vi "AddRows.vi"(6 "GridData":variant, 8 "error in (no error)":errorcluster, 11 "DataGridView in":refnum<class "DataGridView.lvclass">) -> (0 "error out":errorcluster, 3 "DataGridView out":refnum<class "DataGridView.lvclass">)   [LabVIEW 2014, in "DataGridView.lvclass"]
uses:
  DataGridView.lvclass
  DataGridView.lvclass/DataGridView.ctl
  System.Windows.Forms
  GridColumn/GridColumn.lvclass/GridColumn.ctl
  System.Drawing
  GridColumn/Read datatype.vi
  GridColumn/Read Params.vi
  GridColumn/GridColumn.lvclass
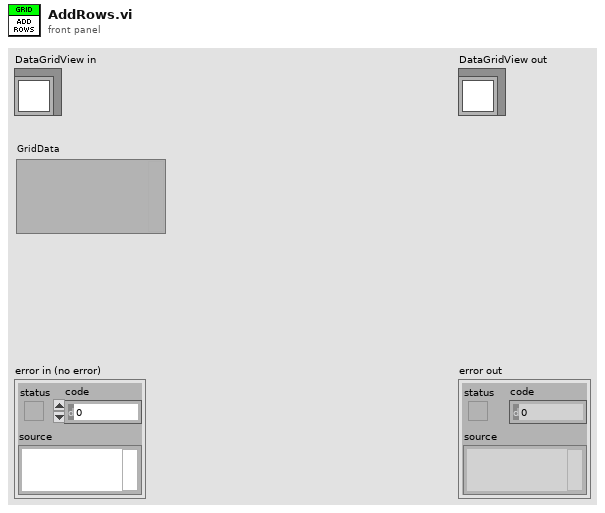
[diagram p1: front panel]
types:
  T1 = enum16{"string", "image", "link", "check", "combo", "button"}
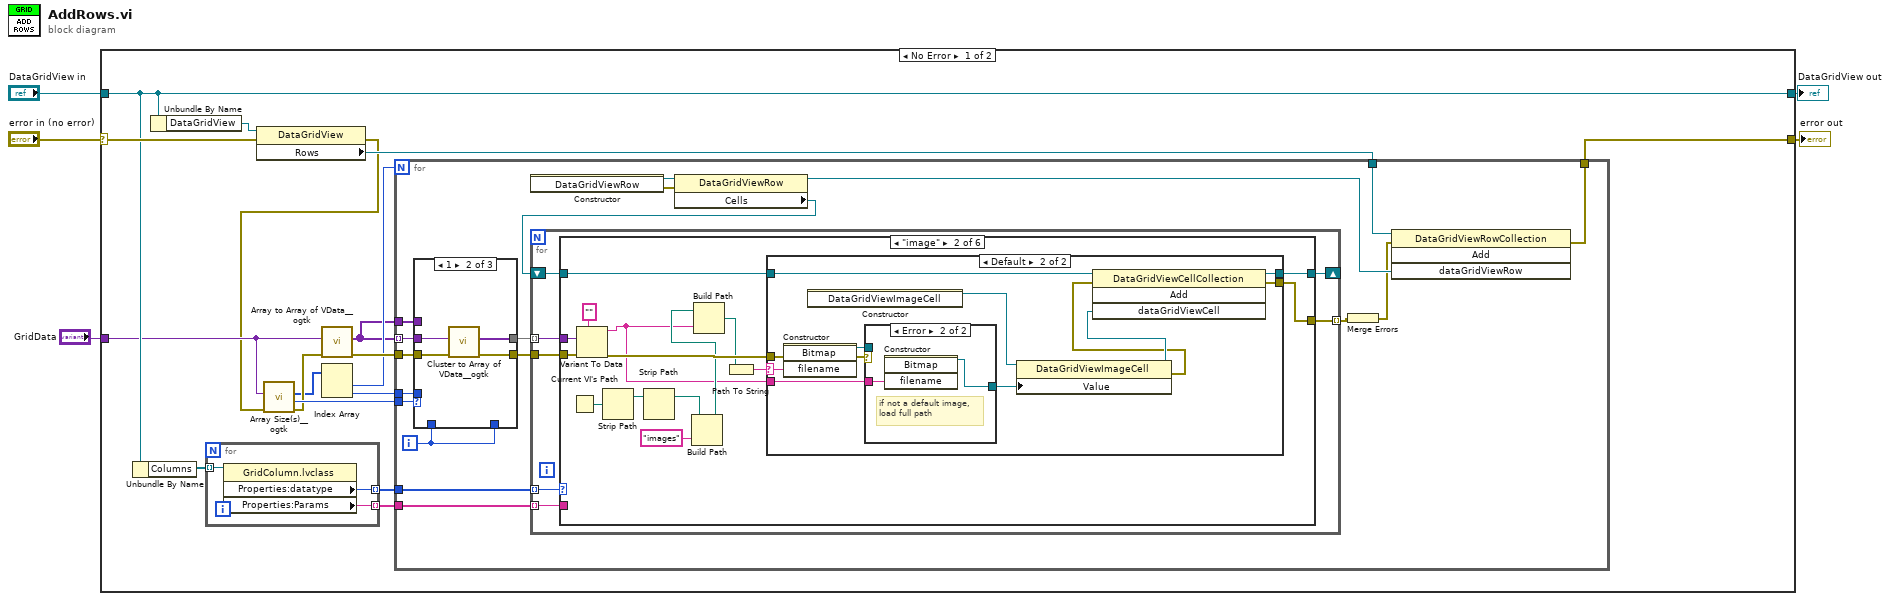
[diagram p0: block diagram]
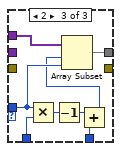
[diagram p3: hidden frame]
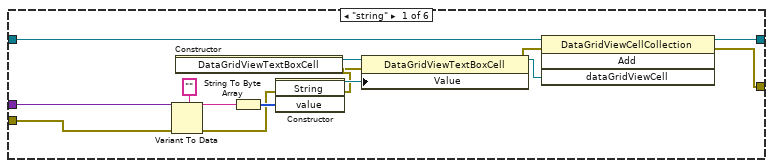
[diagram p4: hidden frame]
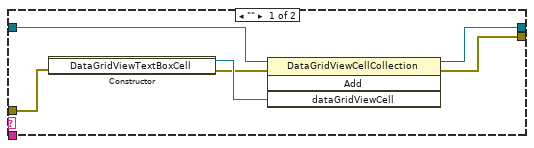
[diagram p5: hidden frame]
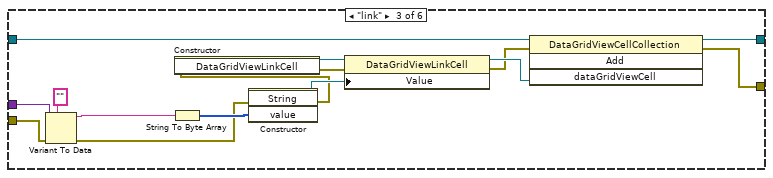
[diagram p7: hidden frame]
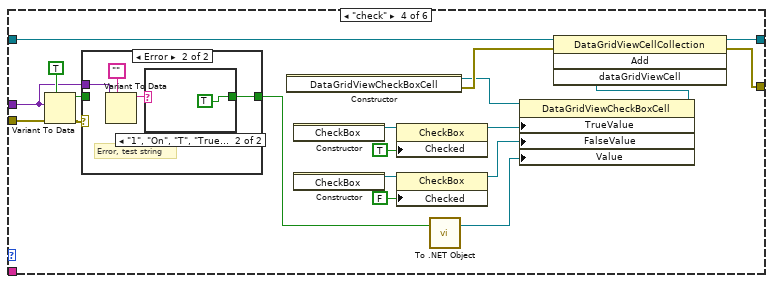
[diagram p8: hidden frame]
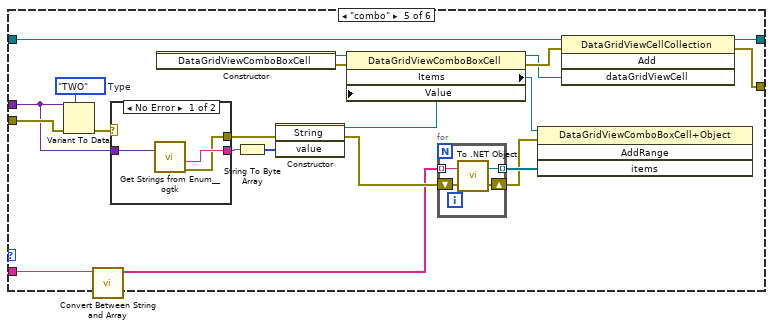
[diagram p11: hidden frame]
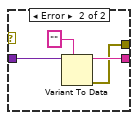
[diagram p12: hidden frame]
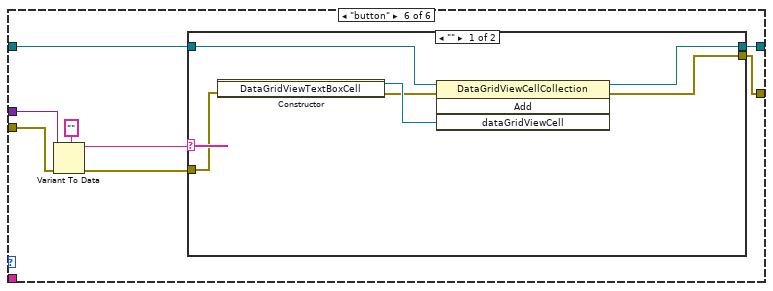
[diagram p13: hidden frame]
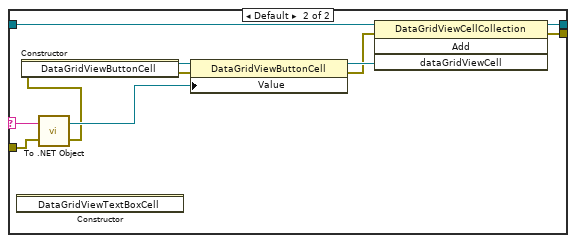
[diagram p14: hidden frame]
diagram:
  n1 = case shown="No Error" "error in (no error)" {
    selector: "error in (no error)" -> [w21 w212]
    tunnel: [w20 w212] -> w4
    tunnel: [w19 w211] -> w2
    tunnel: "DataGridView in" -> [w19 w211]
    tunnel: "GridData" -> [w13 _]
    frame No Error {
      n2 = Unbundle By Name(w19) -> ("Columns"=w18:refnum<class "GridColumn.lvclass">[])
      n3 = Unbundle By Name(w19) -> ("DataGridView"=w22:refnum<k24>)
      n4 = for {
        tunnel: w18 -> [w210] mode=indexing
        tunnel: [w209] -> w17 mode=indexing
        tunnel: [w208] -> w15 mode=indexing
        n5 = property class="GridColumn.lvclass"(reference=w210) -> ("Properties:datatype"=w209:T1, "Properties:Params"=w208:string)  [unwired: 1 in, 2 out]
      }
      n6 = property class="DataGridView"(reference=w22, error in=w21) -> (error out=w10:errorcluster, "Rows"=w16:refnum<k24>)  [unwired: 1 out]
      n7 = call <userlib>:"Array Size(s)__ogtk.vi"("error in (no error)"=w10, "Array"=w13) -> ("error out"=w12:errorcluster, "N dims"=w14:u32, "Size(s)"=w9:u32[])  [unwired: 7 in]
      n8 = call <userlib>:"Array to Array of VData__ogtk.vi"("error in (no error)"=w12, "MultiD Array"=w13) -> ("error out"=w11:errorcluster, "1D Array of Variants"=w6:variant[])  [unwired: 8 in]
      n9 = Index Array(array=w9) -> (element #1=w8:u32, element #2=w7:u32)  [unwired: 2 in]
      n10 = for {
        N: w8 -> [_]
        tunnel: [w40] -> w20
        tunnel: w17 -> [w39]
        tunnel: w16 -> [w33]
        tunnel: w15 -> [w32]
        tunnel: w6 -> [w29] mode=indexing
        tunnel: w14 -> [w28]
        tunnel: w11 -> [w26]
        tunnel: w7 -> [w25]
        tunnel: w6 -> [w23]
        i -> [w24]
        n11 = case shown="1" w28 {
          tunnel: [_ w42 _] -> w30
          tunnel: w29 -> [_ w44 _]
          tunnel: [_ w41 w47] -> w27
          tunnel: w26 -> [_ w43 _]
          tunnel: w25 -> [_ _ w52]
          tunnel: w24 -> [_ _ w51]
          tunnel: w24 -> [_ _ w49]
          tunnel: w23 -> [_ _ w46]
          frame Default {
          }
          frame 1 {
            n12 = call <userlib>:"Cluster to Array of VData__ogtk.vi"("error in (no error)"=w43, "Cluster"=w44) -> ("error out"=w42:errorcluster, "Array of VData"=w41:variant[])  [unwired: 8 in]
          }
          frame 2 {
            n13 = Multiply(x=w52, y=w51) -> (x*y=w50:u32)
            n14 = Decrement(x=w50) -> (x-1=w45:u32)
            n15 = Add(x=w45, y=w49) -> (x+y=w48:u32)
            n16 = Array Subset(array=w46, index=w48, length=w52) -> (w47:variant[])
          }
        }
        n17 = constructor class="DataGridViewRow"() -> (reference out=w37:refnum<k24>, error out=w38:errorcluster)  [unwired: 3 in, 1 out]
        n18 = property class="DataGridViewRow"(reference=w37, error in=w38) -> (reference out=w36:refnum<k24>, "Cells"=w31:refnum<k24>)  [unwired: 1 out]
        n19 = for {
          tunnel: w27 -> [w58] mode=indexing
          tunnel: w39 -> [w59] mode=indexing
          shift-right: [w56] -> _
          shift-left: w31 -> [w57]
          tunnel: w30 -> [w55]
          tunnel: [w54] -> w35 mode=indexing
          tunnel: w32 -> [w53] mode=indexing
          n20 = case shown="\"image\"" w59 {
            tunnel: w58 -> [w74 w84 w125 w126 w156 w185]
            tunnel: w57 -> [w73 w89 w118 w143 w171 w190]
            tunnel: [w72 w88 w116 w142 w170 w189] -> w56
            tunnel: w55 -> [w71 w85 w112 w140 w164 w186]
            tunnel: [w70 w87 w114 w141 w167 w188] -> w54
            tunnel: w53 -> [_ _ _ _ w153 _]
            frame "string" {
              n21 = Variant To Data(error in=w71, type="", Variant=w74) -> (data=w67:string, error out=w63:errorcluster)
              n22 = String To Byte Array(string=w67) -> (unsigned byte array=w68:u8[])
              n23 = constructor class="String"(error in=w63, "value"=w68) -> (reference out=w65:refnum<k24>, error out=w61:errorcluster)  [unwired: 2 in, 2 out]
              n24 = constructor class="DataGridViewTextBoxCell"(error in=w61) -> (reference out=w66:refnum<k24>, error out=w60:errorcluster)  [unwired: 2 in, 1 out]
              n25 = property class="DataGridViewTextBoxCell"(reference=w66, error in=w60, "Value"=w65) -> (reference out=w64:refnum<k24>, error out=w62:errorcluster)
              n26 = invoke class="DataGridViewCellCollection" method="Add"(reference=w73, error in=w62, "dataGridViewCell"=w64) -> (reference out=w72:refnum<k24>, error out=w70:errorcluster)  [unwired: 1 in, 2 out]
            }
            frame "image" {
              n27 = Current VI's Path() -> (path=w81:path)
              n28 = Variant To Data(error in=w85, type="", Variant=w84) -> (data=w75:string, error out=w83:errorcluster)
              n29 = Strip Path(path=w81) -> (stripped path=w80:path)  [unwired: 1 out]
              n30 = Strip Path(path=w80) -> (stripped path=w78:path)  [unwired: 1 out]
              n31 = Build Path(base path=w78, name or relative path="images") -> (appended path=w77:path)
              n32 = Build Path(base path=w77, name or relative path=w75) -> (appended path=w76:path)
              n33 = Path To String(path=w76) -> (string=w82:string)
              n34 = case shown="Default" w82 {
                selector: w82 -> [_ w100]
                tunnel: w89 -> [w93 w107]
                tunnel: [w92 w106] -> w88
                tunnel: [w91 w105] -> w87
                tunnel: w83 -> [w90 w104]
                tunnel: w75 -> [_ w98]
                frame "" {
                  n35 = constructor class="DataGridViewTextBoxCell"(error in=w90) -> (reference out=w95:refnum<k24>, error out=w94:errorcluster)  [unwired: 2 in, 1 out]
                  n36 = invoke class="DataGridViewCellCollection" method="Add"(reference=w93, error in=w94, "dataGridViewCell"=w95) -> (reference out=w92:refnum<k24>, error out=w91:errorcluster)  [unwired: 1 in, 2 out]
                }
                frame Default {
                  n37 = constructor class="Bitmap"(error in=w104, "filename"=w100) -> (reference out=w96:refnum<k24>, error out=w99:errorcluster)  [unwired: 2 in, 2 out]
                  n38 = constructor class="DataGridViewImageCell"() -> (reference out=w102:refnum<k24>)  [unwired: 3 in, 2 out]
                  n39 = case shown="Error" w99 {
                    tunnel: w98 -> [_ w110]
                    tunnel: [w108 w109] -> w97
                    tunnel: w96 -> [w108 _]
                    frame No Error {
                      # "Used when a filename is given."
                    }
                    frame Error {
                      # "if not a default image,\nload full path"
                      n40 = constructor class="Bitmap"("filename"=w110) -> (reference out=w109:refnum<k24>)  [unwired: 3 in, 3 out]
                    }
                  }
                  n41 = property class="DataGridViewImageCell"(reference=w102, "Value"=w97) -> (reference out=w103:refnum<k24>, error out=w101:errorcluster)  [unwired: 1 in]
                  n42 = invoke class="DataGridViewCellCollection" method="Add"(reference=w107, error in=w101, "dataGridViewCell"=w103) -> (reference out=w106:refnum<k24>, error out=w105:errorcluster)  [unwired: 1 in, 2 out]
                }
              }
            }
            frame "link" {
              n43 = Variant To Data(error in=w112, type="", Variant=w125) -> (data=w122:string, error out=w113:errorcluster)
              n44 = String To Byte Array(string=w122) -> (unsigned byte array=w123:u8[])
              n45 = constructor class="String"(error in=w113, "value"=w123) -> (reference out=w121:refnum<k24>, error out=w111:errorcluster)  [unwired: 2 in, 2 out]
              n46 = constructor class="DataGridViewLinkCell"(error in=w111) -> (reference out=w119:refnum<k24>, error out=w120:errorcluster)  [unwired: 2 in, 1 out]
              n47 = property class="DataGridViewLinkCell"(reference=w119, error in=w120, "Value"=w121) -> (reference out=w117:refnum<k24>, error out=w115:errorcluster)
              n48 = invoke class="DataGridViewCellCollection" method="Add"(reference=w118, error in=w115, "dataGridViewCell"=w117) -> (reference out=w116:refnum<k24>, error out=w114:errorcluster)  [unwired: 1 in, 2 out]
            }
            frame "check" {
              n49 = Variant To Data(error in=w140, type=TRUE, Variant=w126) -> (data=w128:bool, error out=w129:errorcluster)
              n50 = case shown="Error" w129 {
                tunnel: w128 -> [w145 _]
                tunnel: [w145 w146] -> w127
                tunnel: w126 -> [_ w147]
                frame No Error {
                }
                frame Error {
                  # "Error, test string"
                  n51 = Variant To Data(type="", Variant=w147) -> (data=w148:string)  [unwired: 1 in, 1 out]
                  n52 = case shown="\"1\", \"On\", \"T\", \"True\", \"Y\"" w148 {
                    tunnel: [_ TRUE] -> w146
                    frame Default {
                    }
                    frame "1", "On", "T", "True", "Y" {
                    }
                  }
                }
              }
              n53 = constructor class="DataGridViewCheckBoxCell"() -> (reference out=w138:refnum<k24>, error out=w139:errorcluster)  [unwired: 3 in, 1 out]
              n54 = constructor class="CheckBox"() -> (reference out=w136:refnum<k24>)  [unwired: 3 in, 2 out]
              n55 = constructor class="CheckBox"() -> (reference out=w132:refnum<k24>)  [unwired: 3 in, 2 out]
              n56 = property class="CheckBox"(reference=w136, "Checked"=TRUE) -> (reference out=w135:refnum<k24>)  [unwired: 1 in, 1 out]
              n57 = property class="CheckBox"(reference=w132, "Checked"=FALSE) -> (reference out=w131:refnum<k24>)  [unwired: 1 in, 1 out]
              n58 = call <vilib>:"To .NET Object.vi"("anything"=w127) -> (".NET object"=w130:refnum<k24>)  [unwired: 1 in, 1 out]
              n59 = property class="DataGridViewCheckBoxCell"(reference=w138, "TrueValue"=w135, "FalseValue"=w131, "Value"=w130) -> (reference out=w137:refnum<k24>)  [unwired: 1 in, 1 out]
              n60 = invoke class="DataGridViewCellCollection" method="Add"(reference=w143, error in=w139, "dataGridViewCell"=w137) -> (reference out=w142:refnum<k24>, error out=w141:errorcluster)  [unwired: 1 in, 2 out]
            }
            frame "combo" {
              w163 = enum16{"ONE", "TWO", "THREE"}."TWO"  # Type
              n61 = Variant To Data(error in=w164, type=w163, Variant=w156) -> (error out=w160:errorcluster)  [unwired: 1 out]
              n62 = call "Convert Between String and Array.vi"("String"=w153) -> ("String Array"=w152:string[])  [unwired: 9 in, 1 out]
              n63 = case shown="No Error" w160 {
                tunnel: [w173 w177] -> w159
                tunnel: w156 -> [w174 w176]
                tunnel: [w172 w175] -> w155
                frame No Error {
                  n64 = call <userlib>:"Get Strings from Enum__ogtk.vi"("Enum"=w174) -> ("error out"=w172:errorcluster, "String Value"=w173:string)  [unwired: 7 in, 2 out]
                }
                frame Error {
                  n65 = Variant To Data(type="", Variant=w176) -> (data=w177:string, error out=w175:errorcluster)  [unwired: 1 in]
                }
              }
              n66 = constructor class="DataGridViewComboBoxCell"() -> (reference out=w166:refnum<k24>, error out=w169:errorcluster)  [unwired: 3 in, 1 out]
              n67 = String To Byte Array(string=w159) -> (unsigned byte array=w158:u8[])
              n68 = constructor class="String"(error in=w155, "value"=w158) -> (reference out=w151:refnum<k24>, error out=w154:errorcluster)  [unwired: 2 in, 2 out]
              n69 = property class="DataGridViewComboBoxCell"(reference=w166, error in=w169, "Value"=w151) -> (reference out=w165:refnum<k24>, error out=w168:errorcluster, "Items"=w157:refnum<k24>)
              n70 = for {
                tunnel: [w182] -> w162 mode=indexing
                tunnel: w152 -> [w181] mode=indexing
                shift-right: [w180] -> w161
                shift-left: w154 -> [w179]
                n71 = call <vilib>:"To .NET Object.vi"("error in (no error)"=w179, "anything"=w181) -> ("error out"=w180:errorcluster, ".NET object"=w182:refnum<k24>)
              }
              n72 = invoke class="DataGridViewComboBoxCell+Object" method="AddRange"(reference=w157, error in=w161, "items"=w162) -> ()  [unwired: 1 in, 4 out]
              n73 = invoke class="DataGridViewCellCollection" method="Add"(reference=w171, error in=w168, "dataGridViewCell"=w165) -> (reference out=w170:refnum<k24>, error out=w167:errorcluster)  [unwired: 1 in, 2 out]
            }
            frame "button" {
              n74 = Variant To Data(error in=w186, type="", Variant=w185) -> (data=w183:string, error out=w184:errorcluster)
              n75 = case shown="\"\"" w183 {
                selector: w183 -> [_ w197]
                tunnel: w190 -> [w196 w207]
                tunnel: [w195 w206] -> w189
                tunnel: [w193 w205] -> w188
                tunnel: w184 -> [w191 w199]
                frame "" {
                  n76 = constructor class="DataGridViewTextBoxCell"(error in=w191) -> (reference out=w194:refnum<k24>, error out=w192:errorcluster)  [unwired: 2 in, 1 out]
                  n77 = invoke class="DataGridViewCellCollection" method="Add"(reference=w196, error in=w192, "dataGridViewCell"=w194) -> (reference out=w195:refnum<k24>, error out=w193:errorcluster)  [unwired: 1 in, 2 out]
                }
                frame Default {
                  n78 = constructor class="DataGridViewTextBoxCell"() -> ()  [unwired: 3 in, 3 out]
                  n79 = call <vilib>:"To .NET Object.vi"("error in (no error)"=w199, "anything"=w197) -> ("error out"=w198:errorcluster, ".NET object"=w204:refnum<k24>)
                  n80 = constructor class="DataGridViewButtonCell"(error in=w198) -> (reference out=w203:refnum<k24>, error out=w201:errorcluster)  [unwired: 2 in, 1 out]
                  n81 = property class="DataGridViewButtonCell"(reference=w203, error in=w201, "Value"=w204) -> (reference out=w202:refnum<k24>, error out=w200:errorcluster)
                  n82 = invoke class="DataGridViewCellCollection" method="Add"(reference=w207, error in=w200, "dataGridViewCell"=w202) -> (reference out=w206:refnum<k24>, error out=w205:errorcluster)  [unwired: 1 in, 2 out]
                }
              }
            }
          }
        }
        n83 = Merge Errors(w35) -> (w34:errorcluster)
        n84 = invoke class="DataGridViewRowCollection" method="Add"(reference=w33, error in=w34, "dataGridViewRow"=w36) -> (error out=w40:errorcluster)  [unwired: 1 in, 3 out]
      }
    }
    frame Error {
    }
  }
  "error out" <- w4
  "DataGridView out" <- w2
